vi "Initialize Buffer Converter Component.vi"(8 "error in (no error)":errorcluster, 9 "Plugin Configuration":refnum<class "Plugin Configuration.lvclass">, 10 "Components":refnum<class "Component.lvclass">[](array[class]), 11 "Transceiver Thread in":refnum<class "Transceiver Thread.lvclass">) -> (0 "error out":errorcluster, 3 "Transceiver Thread out":refnum<class "Transceiver Thread.lvclass">)   [LabVIEW 2020, in "DSF Core.lvlib" / "Transceiver Thread.lvclass"]
uses:
  Transceiver Thread.lvclass
  Thread.lvclass
  Buffer Converter/Buffer Converter.lvclass
  C:/Users/nitest/Desktop/Git/niveristand-data-sharing-framework-custom-device/Source/Core/Classes/Thread/Plugin/Plugin Thread.lvclass
  C:/Users/nitest/Desktop/Git/niveristand-data-sharing-framework-custom-device/Source/Core/Classes/Thread/Thread.lvclass
  C:/Users/nitest/Desktop/Git/niveristand-data-sharing-framework-custom-device/Source/Core/Classes/Thread/Plugin/Transceiver/Transceiver Thread.lvclass
  Component/Component.lvclass
  Configuration/Core/Plugin/Plugin Configuration.lvclass
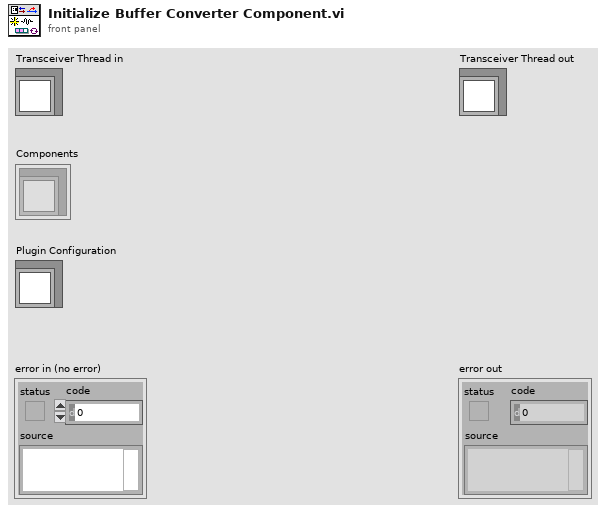
[diagram p1: front panel]
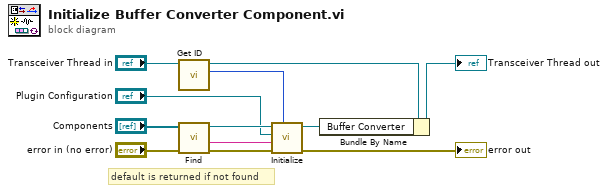
[diagram p0: block diagram]
diagram:
  # "default is returned if not found"
  n1 = call "Get ID.vi"("Thread in"="Transceiver Thread in") -> ("ID"=w1:i32, "Thread out"=w12:refnum<class "Transceiver Thread.lvclass">)  [unwired: 9 in]
  n2 = call "Find.vi"("error in (no error)"="error in (no error)", "Components"="Components") -> ("error out"=w6:errorcluster, "component name"=w3:string, "Buffer Converter"=w7:refnum<class "Buffer Converter.lvclass">)  [unwired: 6 in, 1 out]
  n3 = call-dynamic "Initialize.vi"("thread ID"=w1, "error in (no error)"=w6, "component name"=w3, "Plugin Configuration"="Plugin Configuration", "Buffer Converter in"=w7) -> ("error out"=→"error out":errorcluster, "Buffer Converter out"=w4:refnum<class "Buffer Converter.lvclass">)  [unwired: 5 in]
  n4 = Bundle By Name(cluster=w12, "Buffer Converter"=w4) -> (→"Transceiver Thread out":refnum<class "Transceiver Thread.lvclass">)
